vi "EmirhanLabWiew.vi"() -> ()   [LabVIEW 2021]
uses:
  Program Files (x86)/National Instruments/LabVIEW 2021/examples/Instrument IO/Serial/support/Serial - Settings.ctl
  <vilib>/Utility/file.llb/Write Delimited Spreadsheet (string).vi
  <vilib>/Instr/_visa.llb/VISA Configure Serial Port (Instr).vi
  <vilib>/Utility/file.llb/Write Delimited Spreadsheet (DBL).vi
panel:
  out "appended array":dbl[](array[numeric])
  out "Array":string[](array[string])
  in  "file path (dialog if empty) 2":path
  out "JoyStick-Y":dbl(graph)
  out "Y":dbl
  out "JoyStick-X":dbl(graph)
  out "X":dbl
  out "SerçeParmak Chart":dbl(graph)
  out "SerçeParmak":dbl
  out "YüzükParmak Chart":dbl(graph)
  out "YüzükParmak":dbl
  out "OrtaParmak Chart":dbl(graph)
  out "OrtaParmak":dbl
  out "İsaretParmak Chart":dbl(graph)
  out "İsaretParmak":dbl
  out "BasParmak Chart":dbl(graph)
  out "BasParmak":dbl
  in  "stop":bool
  in  "Serial Settings":T1={"baud rate"=9600, "data bits"=8, "parity"=enum."None", "stop bits"=10, "flow control"=0} {"flow control" items=["None"=0, "XON/XOFF"=1, "RTS/CTS"=2, "DTR/DSR"=4]; "stop bits" items=["1.0"=10, "1.5"=15, "2.0"=20]; "data bits" min=5 max=8 step=1; "baud rate" items=["75"=75, "110"=110, "134"=134, "150"=150, "300"=300, "600"=600, "1200"=1200, "1800"=1800, "2400"=2400, "4800"=4800, "7200"=7200, "115200"=9600, "14400"=14400, "19200"=19200, "28800"=28800, "38400"=38400, "56000"=56000, "57600"=57600, "115200"=115200, "128000"=128000, "230400"=230400]}
  out "bytes read":u32
  in  "VISA resource name":refnum<visa-resource-name>="COM1"
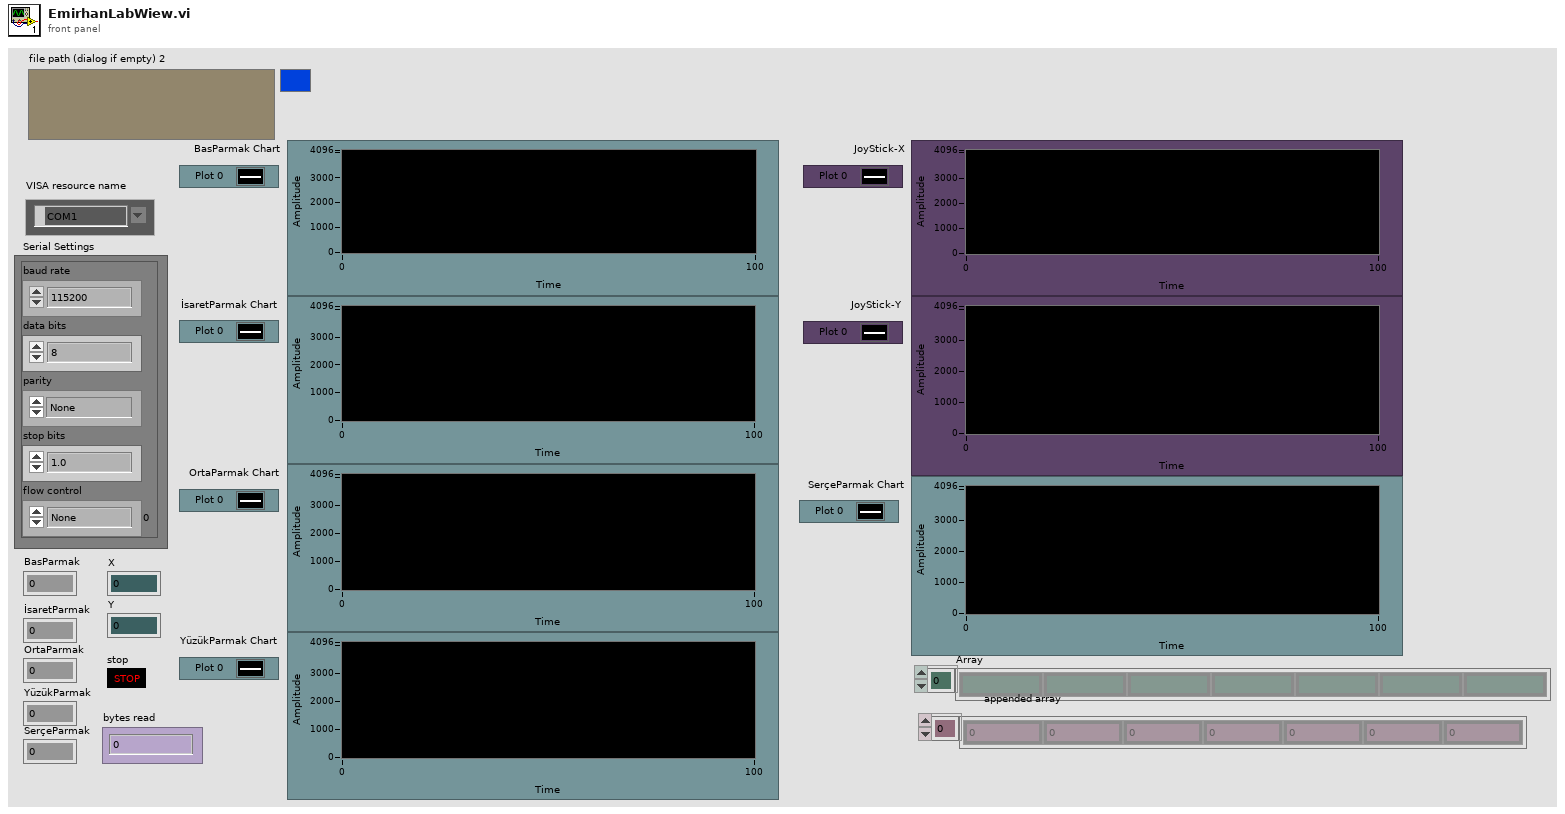
[diagram p1: front panel]
types:
  T1 = typedef "Serial - Settings.ctl" = cluster{"baud rate":u32, "data bits":u16, "parity":enum16{"None", "Odd", "Even", "Mark", "Space"}, "stop bits":u16, "flow control":u16}
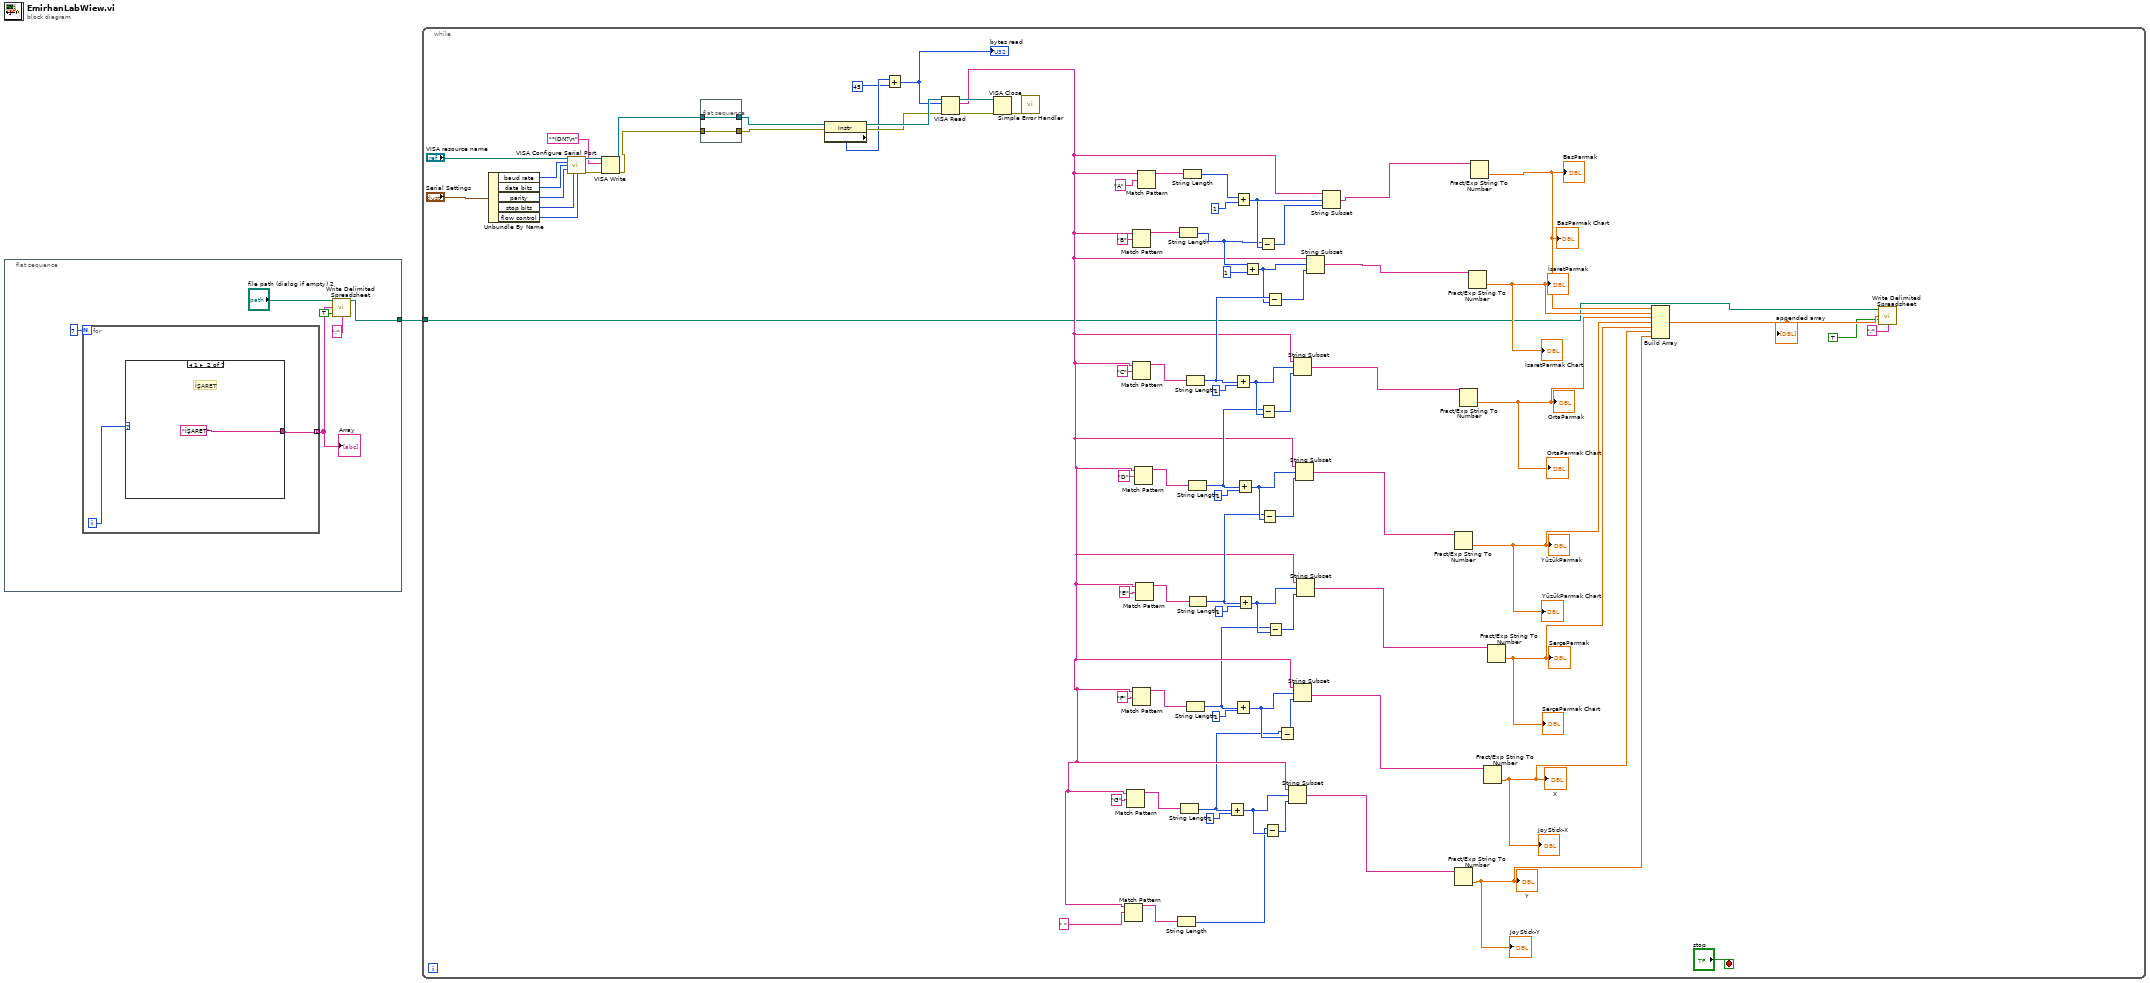
[diagram p0: block diagram]
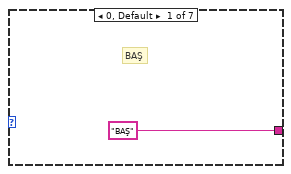
[diagram p2: hidden frame]
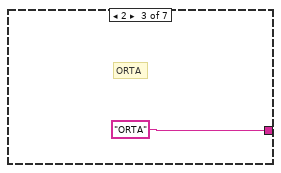
[diagram p3: hidden frame]
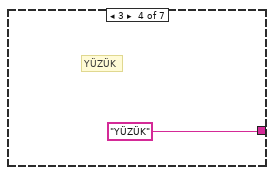
[diagram p4: hidden frame]
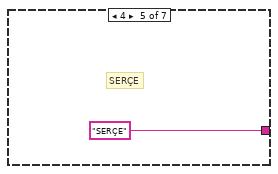
[diagram p5: hidden frame]
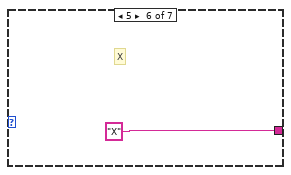
[diagram p6: hidden frame]
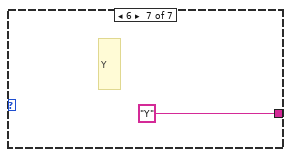
[diagram p7: hidden frame]
diagram:
  n1 = flat-sequence {
    tunnel: [w5] -> w1
    frame #0 {
      n2 = for {
        N: 7 -> [_]
        tunnel: [w8] -> w3 mode=indexing
        i -> [w9]
        n3 = case shown="1" w9 {
          tunnel: ["BAŞ" "İŞARET" "ORTA" "YÜZÜK" "SERÇE" "X" "Y"] -> w8
          frame 0, Default {
            # "BAŞ"
          }
          frame 1 {
            # "İŞARET"
          }
          frame 2 {
            # "ORTA"
          }
          frame 3 {
            # "YÜZÜK"
          }
          frame 4 {
            # "SERÇE"
          }
          frame 5 {
            # "X"
          }
          frame 6 {
            # "Y"
          }
        }
      }
      "Array" <- w3
      n4 = call-poly <vilib>:"Write Delimited Spreadsheet.vi"("file path (dialog if empty)"="file path (dialog if empty) 2", "1D data"=w3, "append to file? (new file:F)"=TRUE, "delimiter (\\t)"=";" ("delimiter (\\t)")) -> ("new file path (Not A Path if cancelled)"=w5:path)  [unwired: 10 in, 1 out]
    }
  }
  n5 = while {
    tunnel: w1 -> [w20]
    stop <- "stop" stop-if-true
    n6 = Unbundle By Name("Serial Settings") -> ("baud rate"=w36:u32, "data bits"=w37:u16, "parity"=w38:enum16{"None", "Odd", "Even", "Mark", "Space"}, "stop bits"=w39:u16, "flow control"=w40:u16)
    n7 = call-poly "VISA Configure Serial Port"("VISA resource name"="VISA resource name", "baud rate (115200)"=w36, "data bits (8)"=w37, "parity (0:none)"=w38, "stop bits (10: 1 bit)"=w39, "flow control (0:none)"=w40) -> ("VISA resource name out"=w34:refnum<visa-resource-name>, "error out"=w33:errorcluster)  [unwired: 3 in, 5 out]
    n8 = VISA Write(VISA resource name=w34, write buffer="*IDN?\n" ("Command"), error in (no error)=w33) -> (VISA resource name out=w29:refnum<visa-resource-name>, error out=w30:errorcluster)  [unwired: 1 out]
    n9 = flat-sequence {
      tunnel: w30 -> [w105]
      tunnel: [w105] -> w100
      tunnel: w29 -> [w104]
      tunnel: [w104] -> w99
      frame #0 {
      }
    }
    n10 = property class="Instr"(reference=w99, error in=w100) -> (reference out=w98:refnum<visa-resource-name>, error out=w97:errorcluster, "Serial Settings:Number of Bytes at Serial Port"=w43:u32)
    n11 = Add(x=w43, y=45) -> (x+y=w41:u32)
    "bytes read" <- w41
    n12 = VISA Read(VISA resource name=w98, byte count=w41, error in (no error)=w97) -> (VISA resource name out=w102:refnum<visa-resource-name>, read buffer=w61:string, error out=w103:errorcluster)  [unwired: 1 out]
    n13 = VISA Close(VISA resource name=w102, error in (no error)=w103) -> (error out=w101:errorcluster)
    n14 = call <vilib>:"Simple Error Handler.vi"("error in (no error)"=w101) -> ()  [unwired: 1 in, 8 out]
    n15 = Match Pattern(string=w61, regular expression=" ") -> (before substring=w62:string)  [unwired: 1 in, 3 out]
    n16 = Match Pattern(string=w61, regular expression="G") -> (before substring=w65:string)  [unwired: 1 in, 3 out]
    n17 = Match Pattern(string=w61, regular expression="B") -> (before substring=w92:string)  [unwired: 1 in, 3 out]
    n18 = Match Pattern(string=w61, regular expression="C") -> (before substring=w89:string)  [unwired: 1 in, 3 out]
    n19 = Match Pattern(string=w61, regular expression="F") -> (before substring=w68:string)  [unwired: 1 in, 3 out]
    n20 = Match Pattern(string=w61, regular expression="D") -> (before substring=w80:string)  [unwired: 1 in, 3 out]
    n21 = Match Pattern(string=w61, regular expression="E") -> (before substring=w77:string)  [unwired: 1 in, 3 out]
    n22 = Match Pattern(string=w61, regular expression="A") -> (before substring=w82:string)  [unwired: 1 in, 3 out]
    n23 = String Length(string=w62) -> (length=w54:i32)
    n24 = String Length(string=w92) -> (length=w85:i32)
    n25 = String Length(string=w65) -> (length=w56:i32)
    n26 = String Length(string=w82) -> (length=w94:i32)
    n27 = String Length(string=w89) -> (length=w84:i32)
    n28 = String Length(string=w68) -> (length=w58:i32)
    n29 = String Length(string=w80) -> (length=w71:i32)
    n30 = String Length(string=w77) -> (length=w70:i32)
    n31 = Add(x=w56, y=1) -> (x+y=w55:i32)
    n32 = Add(x=w84, y=1) -> (x+y=w73:i32)
    n33 = Add(x=w58, y=1) -> (x+y=w57:i32)
    n34 = Add(x=w94, y=1) -> (x+y=w91:i32)
    n35 = Add(x=w71, y=1) -> (x+y=w72:i32)
    n36 = Add(x=w70, y=1) -> (x+y=w59:i32)
    n37 = Add(x=w85, y=1) -> (x+y=w83:i32)
    n38 = Subtract(x=w85, y=w91) -> (x-y=w51:i32)
    n39 = Subtract(x=w71, y=w73) -> (x-y=w74:i32)
    n40 = Subtract(x=w70, y=w72) -> (x-y=w75:i32)
    n41 = Subtract(x=w54, y=w55) -> (x-y=w53:i32)
    n42 = Subtract(x=w84, y=w83) -> (x-y=w86:i32)
    n43 = Subtract(x=w58, y=w59) -> (x-y=w60:i32)
    n44 = Subtract(x=w56, y=w57) -> (x-y=w52:i32)
    n45 = String Subset(string=w61, offset (0)=w55, length (rest)=w53) -> (substring=w44:string)
    n46 = String Subset(string=w61, offset (0)=w73, length (rest)=w74) -> (substring=w48:string)
    n47 = String Subset(string=w61, offset (0)=w57, length (rest)=w52) -> (substring=w45:string)
    n48 = String Subset(string=w61, offset (0)=w72, length (rest)=w75) -> (substring=w47:string)
    n49 = String Subset(string=w61, offset (0)=w59, length (rest)=w60) -> (substring=w46:string)
    n50 = String Subset(string=w61, offset (0)=w83, length (rest)=w86) -> (substring=w21:string)
    n51 = String Subset(string=w61, offset (0)=w91, length (rest)=w51) -> (substring=w49:string)
    n52 = Fract/Exp String To Number(string=w47) -> (number=w25:dbl)  [unwired: 3 in, 1 out]
    "YüzükParmak" <- w25
    "YüzükParmak Chart" <- w25
    n53 = Fract/Exp String To Number(string=w44) -> (number=w22:dbl)  [unwired: 3 in, 1 out]
    "Y" <- w22
    "JoyStick-Y" <- w22
    n54 = Fract/Exp String To Number(string=w48) -> (number=w26:dbl)  [unwired: 3 in, 1 out]
    "OrtaParmak" <- w26
    "OrtaParmak Chart" <- w26
    n55 = Fract/Exp String To Number(string=w21) -> (number=w27:dbl)  [unwired: 3 in, 1 out]
    "İsaretParmak" <- w27
    "İsaretParmak Chart" <- w27
    n56 = Fract/Exp String To Number(string=w49) -> (number=w28:dbl)  [unwired: 3 in, 1 out]
    "BasParmak" <- w28
    "BasParmak Chart" <- w28
    n57 = Fract/Exp String To Number(string=w45) -> (number=w23:dbl)  [unwired: 3 in, 1 out]
    "X" <- w23
    "JoyStick-X" <- w23
    n58 = Fract/Exp String To Number(string=w46) -> (number=w24:dbl)  [unwired: 3 in, 1 out]
    "SerçeParmak" <- w24
    "SerçeParmak Chart" <- w24
    n59 = Build Array(w28, w27, w26, w25, w24, w23, w22) -> (w19:dbl[])
    "appended array" <- w19
    n60 = call-poly <vilib>:"Write Delimited Spreadsheet.vi"("file path (dialog if empty)"=w20, "1D data"=w19, "append to file? (new file:F)"=TRUE, "delimiter (\\t)"=";" ("delimiter (\\t)")) -> ()  [unwired: 10 in, 2 out]
  }
